vi "LWXPS_GroupSpineModeStop.vi"(6 "LabVIEW error IN":errorcluster, 7 "Acceleration":dbl, 8 "Group Name":string, 9 "XPS Reference IN":refnum<k24>) -> (0 "LabVIEW error OUT":errorcluster, 1 "XPS Error String":string, 2 "Returned error code":i32, 3 "XPS Reference OUT":refnum<k24>)   [LabVIEW 2014]
uses:
  D:/XPSQ8_LabView_Library/Development/Source/Dll/Newport.XPS.CommandInterface.dll
  Dll/Newport.XPS.CommandInterface.dll
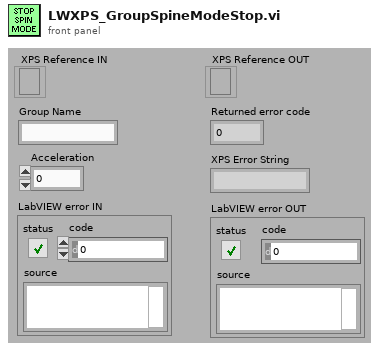
[diagram p1: front panel]
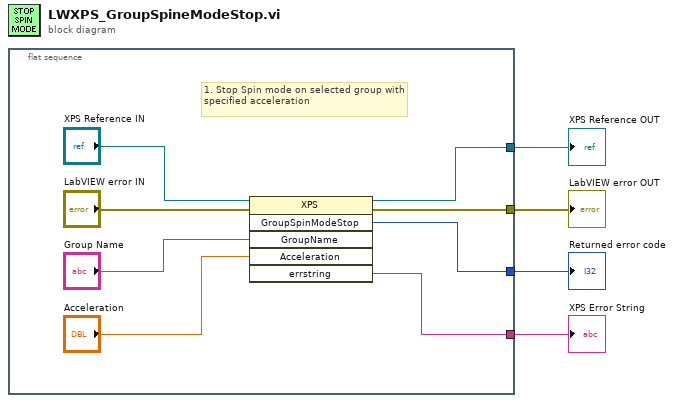
[diagram p0: block diagram]
diagram:
  n1 = flat-sequence {
    tunnel: [w8] -> w4
    tunnel: [w10] -> w3
    tunnel: [w11] -> w2
    tunnel: [w6] -> w1
    frame #0 {
      # "1. Stop Spin mode on selected group with specified acceleration"
      n2 = invoke class="XPS" method="GroupSpinModeStop"(reference="XPS Reference IN", error in="LabVIEW error IN", "GroupName"="Group Name", "Acceleration"="Acceleration") -> (reference out=w8:refnum<k24>, error out=w10:errorcluster, "GroupSpinModeStop"=w11:i32, "errstring"=w6:string)  [unwired: 2 in, 2 out]
    }
  }
  "XPS Reference OUT" <- w4
  "LabVIEW error OUT" <- w3
  "Returned error code" <- w2
  "XPS Error String" <- w1
